vi "Split_String.vi"() -> ()   [LabVIEW 2024]
panel:
  out "offset of match":i32
  out "match + rest of string":string
  out "substring before match":string
  in  "Input String":string
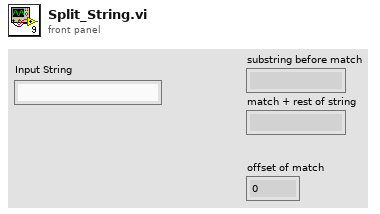
[diagram p1: front panel]
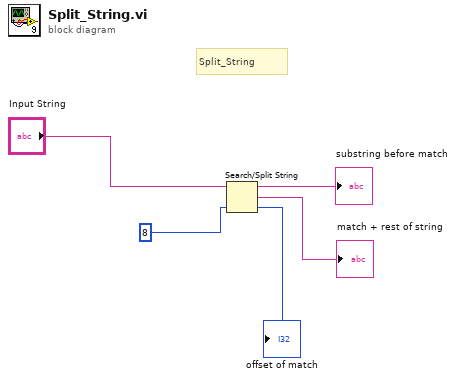
[diagram p0: block diagram]
diagram:
  # "Split_String"
  n1 = Search/Split String(string="Input String", offset (0)=8) -> (substring before match=→"substring before match":string, match + rest of string=→"match + rest of string":string, offset of match=→"offset of match":i32)  [unwired: 1 in]
